vi "Sort moves by minimum incremental travel.vi"(6 "Exclude Array":T1[](array[typedef]) {"Sizes"."Min" format="%#.1f"; "Sizes"."Max" format="%#.1f"}, 7 "moveCostWeighting":sgl[](array[numeric])=[1.0, 1.0, 1.0], 9 "Coordinates to move through":sgl[][](array[numeric]), 11 "huntBestStart?":bool) -> (0 "path-OriginalStart":dbl, 1 "Order-OriginalStart":i32[](array[numeric]), 2 "path-BestStart":dbl, 3 "Order-BestStart":i32[](array[numeric]))   [LabVIEW 2021]
doc: "Sorts moves in order of minimum incremental linear travel distance, starting from the first point in the list."
uses:
  Route mapping/Exclude_cluster.ctl
  Route mapping/Box_size.ctl
  Route mapping/Exclusion_type.ctl
  d4d1eac6-a9c3-ec43-811f-b9ffa0894db1.vi
panel:
  out "pointNum":i32
  out "testNum":i32
  out "startPoint":i32
  out "path-WorstStart":dbl
  out "path-Unsorted":dbl
  # "Solves the TSP   Naively calculates the shortest route through a set of points by choosing the closest next point at each juncture.\nMoveCostWeighting can be used to discourage use of particular axes.\nIf \"HuntBestStart\" is true, solves the TSP works through all possible starting locations, to find best...\n\nIf \"Travel Above Height\" is set, takes account of Up-and-Over and Up-and-Away moves as required (but doesn't deal with \"Exclude Completely\")"
  # "Paul Nathan 02/07/2015\nTCRL 2023-09-23"
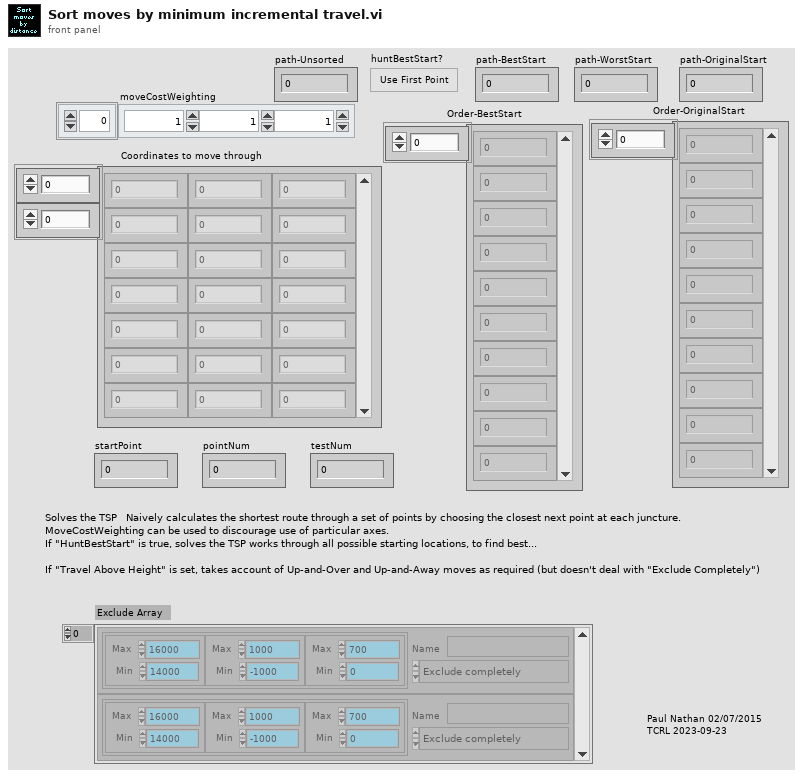
[diagram p1: front panel]
types:
  T1 = typedef "Exclude_cluster.ctl" = cluster{"Sizes":T2, "Name":string, "Exclude Type":T3}
  T2 = typedef "Box_size.ctl" = cluster{"Max":sgl, "Min":sgl}[]
  T3 = typedef "Exclusion_type.ctl" = enum16{"Exclude completely", "Allow only vertical moves"}
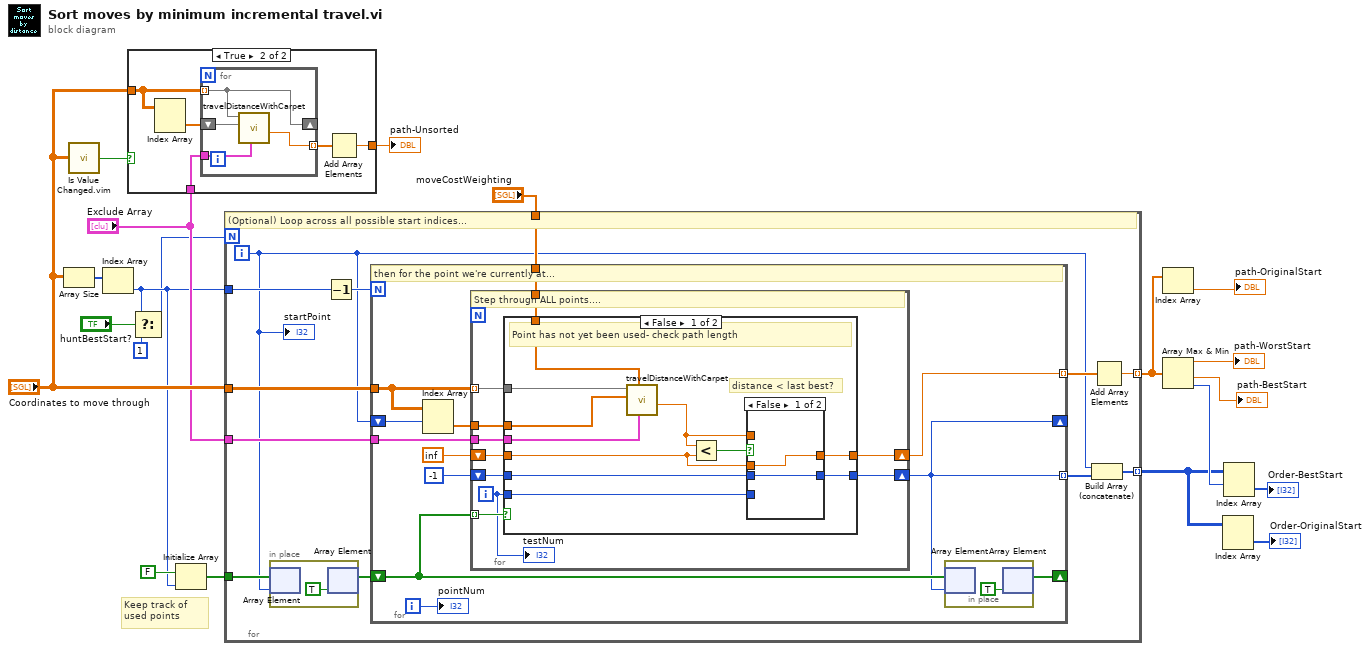
[diagram p0: block diagram]
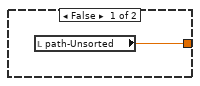
[diagram p4: hidden frame]
diagram:
  # "Keep track of used points"
  n1 = Array Size(array="Coordinates to move through") -> (size(s)=w20:i32[])
  n2 = call "Is Value Changed.vim"("value"="Coordinates to move through") -> ("changed or first call?"=w17:bool)
  n3 = Index Array(array=w20) -> (element=w3:i32)  [unwired: 1 in]
  n4 = case shown="True" w17 {
    tunnel: [w21 w25] -> w19
    tunnel: "Coordinates to move through" -> [_ w23]
    tunnel: "Exclude Array" -> [_ w22]
    frame False {
      n5 = local read "path-Unsorted"() -> (w21:dbl)
    }
    frame True {
      n6 = Index Array(array=w23) -> (element=w24:sgl[])  [unwired: 2 in]
      n7 = for {
        tunnel: w23 -> [w27] mode=indexing
        tunnel: [w30] -> w26 mode=indexing
        shift-right: [w27] -> _
        shift-left: w24 -> [w28]
        tunnel: w22 -> [w29]
        n8 = call "travelDistanceWithCarpet.vi"("Exclude Array"=w29, "pointB"=w28, "pointA"=w27) -> ("distance"=w30:dbl)  [unwired: 7 in, 1 out]
      }
      n9 = Add Array Elements(numeric array=w26) -> (sum=w25:dbl)
    }
  }
  "path-Unsorted" <- w19
  n10 = Select(t=w3, s="huntBestStart?", f=1) -> (s? t:f=w2:i32)
  n11 = Initialize Array(FALSE, w3) -> (w10:bool[])
  n12 = for {
    N: w2 -> [_]
    tunnel: w3 -> [w42]
    tunnel: "Exclude Array" -> [w38]
    tunnel: "Coordinates to move through" -> [w36]
    tunnel: [w35] -> w13 mode=indexing
    tunnel: [w34] -> w8 mode=indexing
    tunnel: w10 -> [w32]
    tunnel: "moveCostWeighting" -> [w33]
    i -> [w31]
    # "(Optional) Loop across all possible start indices..."
    n13 = in-place {
      n14 = in-place-array #1(w32, w31) -> ()  [unwired: 1 out]
      n15 = in-place-array #1(TRUE ("element")) -> (w41:bool[])  [unwired: 1 out]
    }
    n16 = Decrement(x=w42) -> (x-1=w40:i32)
    n17 = for {
      N: w40 -> [_]
      shift-right: [w52] -> _
      shift-left: w41 -> [w53]
      shift-right: [w47] -> _
      shift-left: w31 -> [w48]
      tunnel: [w47] -> w39 mode=indexing
      tunnel: w36 -> [w49]
      tunnel: w38 -> [w46]
      tunnel: [w45] -> w37 mode=indexing
      tunnel: w33 -> [w44]
      i -> [w43]
      # "then for the point we're currently at..."
      n18 = Index Array(array=w49, index (row)=w48) -> (element=w50:sgl[])  [unwired: 1 in]
      n19 = for {
        tunnel: w49 -> [w64] mode=indexing
        tunnel: w53 -> [w62] mode=indexing
        shift-right: [w58] -> w47
        shift-left: -1 -> [w60]
        shift-right: [w57] -> w45
        shift-left: inf ("index (row)") -> [w61]
        tunnel: w50 -> [w63]
        tunnel: w46 -> [w56]
        tunnel: w44 -> [w55]
        i -> [w59]
        # "Step through ALL points...."
        n20 = case shown="False" w62 {
          tunnel: w64 -> [w68 _]
          tunnel: w63 -> [w75 _]
          tunnel: w61 -> [w70 w81]
          tunnel: w60 -> [w69 w80]
          tunnel: w59 -> [w73 _]
          tunnel: [w72 w80] -> w58
          tunnel: [w71 w81] -> w57
          tunnel: w56 -> [w66 _]
          tunnel: w55 -> [w65 _]
          frame False {
            # "distance < last best?"
            # "Point has not yet been used- check path length"
            n21 = call "travelDistanceWithCarpet.vi"("Exclude Array"=w66, "moveCostWeighting"=w65, "pointB"=w75, "pointA"=w68) -> ("distance"=w67:dbl)  [unwired: 6 in, 1 out]
            n22 = Less?(x=w67, y=w70) -> (x < y?=w74:bool)
            n23 = case shown="False" w74 {
              tunnel: w73 -> [_ w79]
              tunnel: [w76 w79] -> w72
              tunnel: [w77 w78] -> w71
              tunnel: w67 -> [_ w78]
              tunnel: w70 -> [w77 _]
              tunnel: w69 -> [w76 _]
              frame False {
              }
              frame True {
              }
            }
          }
          frame True {
            # "(That includes this point itself!)"
            # "Point has already been used..."
          }
        }
        "testNum" <- w59
      }
      n24 = in-place {
        n25 = in-place-array #2(w53, w47) -> ()  [unwired: 1 out]
        n26 = in-place-array #2(TRUE ("element")) -> (w52:bool[])  [unwired: 1 out]
      }
      "pointNum" <- w43
    }
    n27 = Build Array (concatenate)(w31, w39) -> (w34:i32[])
    n28 = Add Array Elements(numeric array=w37) -> (sum=w35:dbl)
    "startPoint" <- w31
  }
  n29 = Index Array(array=w13) -> (element=→"path-OriginalStart":dbl)  [unwired: 1 in]
  n30 = Array Max & Min(array=w13) -> (max value=→"path-WorstStart":dbl, min value=→"path-BestStart":dbl, min index (indices)=w15:i32)  [unwired: 1 out]
  n31 = Index Array(array=w8) -> (element=→"Order-OriginalStart":i32[])  [unwired: 2 in]
  n32 = Index Array(array=w8, index (row)=w15) -> (element=→"Order-BestStart":i32[])  [unwired: 1 in]
